vi "loadSettings.vi"(8 "error in (no error)":errorcluster, 10 "SettingToApply":string, 11 "Model in":refnum<class "Model.lvclass">) -> (0 "error out":errorcluster, 3 "Model out":refnum<class "Model.lvclass">)   [LabVIEW 2016, in "Model.lvclass"]
uses:
  Model.lvclass
  Model.lvclass/Model.ctl
  Boot/Boot.lvclass
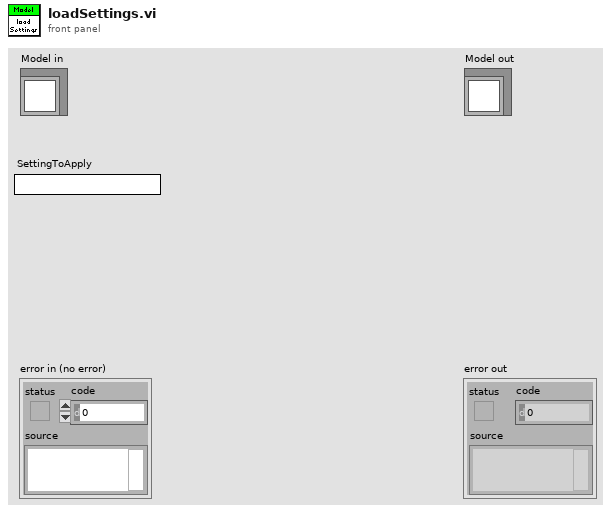
[diagram p1: front panel]
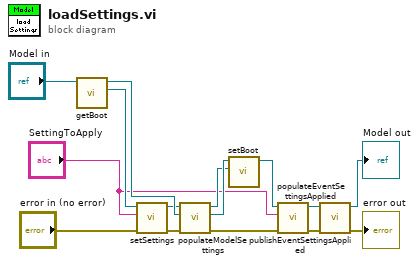
[diagram p0: block diagram]
diagram:
  n1 = call "getBoot.vi"("Model in"="Model in") -> ("Boot"=w13:refnum<class "Boot.lvclass">, "Model out"=w15:refnum<class "Model.lvclass">)  [unwired: 9 in]
  n2 = call "setSettings.vi"("error in (no error)"="error in (no error)", "SettingToApply"="SettingToApply", "Boot in"=w13) -> ("error out"=w11:errorcluster, "Boot out"=w12:refnum<class "Boot.lvclass">)  [unwired: 7 in]
  n3 = call "populateModelSettings.vi"("error in (no error)"=w11, "Model in"=w15, "Boot in"=w12) -> ("error out"=w6:errorcluster, "Model out"=w9:refnum<class "Model.lvclass">, "Boot out"=w8:refnum<class "Boot.lvclass">)  [unwired: 6 in]
  n4 = call "setBoot.vi"("Boot"=w8, "Model in"=w9) -> ("Model out"=w7:refnum<class "Model.lvclass">)  [unwired: 9 in]
  n5 = call "populateEventSettingsApplied.vi"("error in (no error)"=w6, "SettingsApplied"="SettingToApply", "Model in"=w7) -> ("error out"=w3:errorcluster, "Model out"=w4:refnum<class "Model.lvclass">)  [unwired: 7 in]
  n6 = call "publishEventSettingsApplied.vi"("error in (no error)"=w3, "Model in"=w4) -> ("error out"=→"error out":errorcluster, "Model out"=→"Model out":refnum<class "Model.lvclass">)  [unwired: 8 in]
